vi "PH_PPMA_PowerUnit.Calc State PU.vi"(0 "i ref in":refnum<vi>, 5 "error in (no error)":errorcluster) -> (14 "i ref out":refnum<vi>, 19 "error out":errorcluster)   [LabVIEW 2014, in "PH_PPMA_PowerUnit.lvlib"]
doc: "In this VI the state of the PU (running, failure or alarm) is calculated. Depending on the state, several things are done."
uses:
  PH_PPMA_PowerUnit.lvlib
  CSCore/CSSystem/CSSystemLib/CSSystemLib.lvlib
  CSCore/BaseProcess/BaseProcess.lvlib
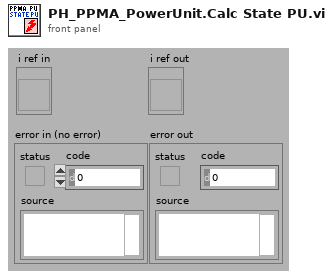
[diagram p1: front panel]
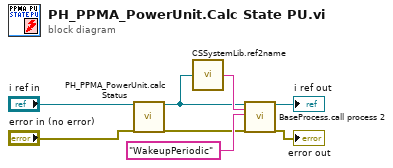
[diagram p0: block diagram]
diagram:
  n1 = call "PH_PPMA_PowerUnit.calc Status.vi"("i ref in"="i ref in", "error in (no error)"="error in (no error)") -> ("i ref out"=w4:refnum<vi>, "error out"=w3:errorcluster)  [unwired: 16 in]
  n2 = call "CSSystemLib.ref2name.vi"("obj refnum"=w4) -> ("name"=w7:string)
  n3 = call "BaseProcess.call process 2.vi"("i ref in"=w4, "Object"=w7, "Selector"="WakeupPeriodic", "error in (no error)"=w3) -> ("i ref out"=→"i ref out":refnum<vi>, "error out"=→"error out":errorcluster)  [unwired: 14 in]
